vi "WFInvertA.vi"(4 "error in (no error)":errorcluster, 7 "Waveform In":waveform(dbl)={"t0"=timestamp(0 s since 1904-01-01), "dt"=0.0, "Y"=[]}) -> (0 "error out":errorcluster, 3 "Waveform Out":waveform(dbl))   [LabVIEW 2013]
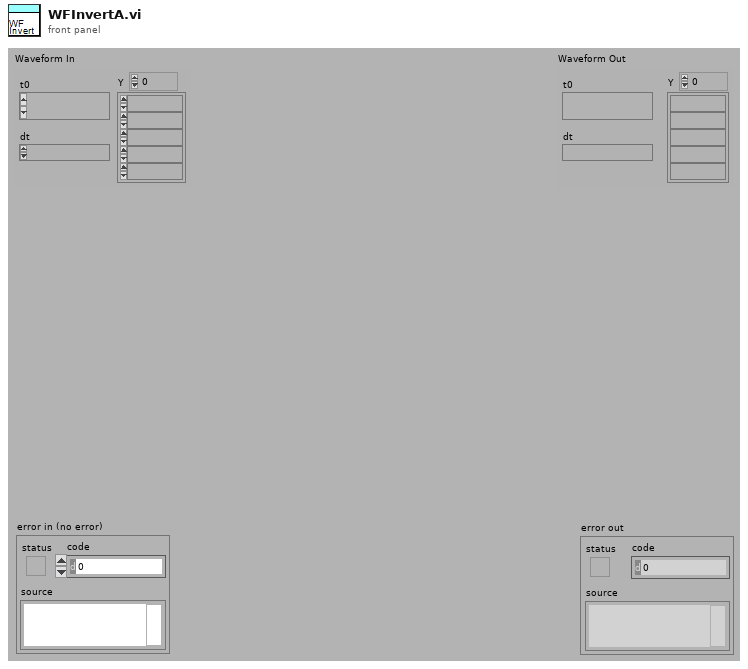
[diagram p1: front panel]
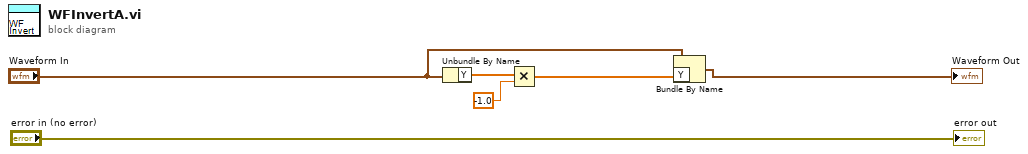
[diagram p0: block diagram]
diagram:
  n1 = Unbundle By Name("Waveform In") -> ("Y"=w5:dbl[])
  n2 = Multiply(x=w5, y=-1.0) -> (x*y=w3:dbl[])
  n3 = Bundle By Name(cluster="Waveform In", "Y"=w3) -> (→"Waveform Out":waveform(dbl))
  "error out" <- "error in (no error)"
